vi "CurrentSwitchValues_GlobalVariable.vi"() -> ()   [LabVIEW 2018]
panel:
  out "Current Reactor":dbl
  in  "Reactor RR Array":dbl[](array[numeric])
  out "Refresh Ratio Reactor 8":dbl
  out "Refresh Ratio Reactor 7":dbl
  out "Refresh Ratio Reactor 6":dbl
  out "Refresh Ratio Reactor 5":dbl
  out "Refresh Ratio Reactor 4":dbl
  out "Refresh Ratio Reactor 3":dbl
  out "Refresh Ratio Reactor 2":dbl
  out "Refresh Ratio Reactor 1":dbl
  out "Refresh Ratio Average":dbl
  out "Number of Inflow Steps Used During Calibration":dbl
  out "30":bool
  out "29":bool
  out "28":bool
  out "27":bool
  out "26":bool
  out "25":bool
  out "24":bool
  out "23":bool
  out "22":bool
  out "21":bool
  out "20":bool
  out "19":bool
  out "18":bool
  out "17":bool
  out "16":bool
  out "15":bool
  out "14":bool
  out "13":bool
  out "12":bool
  out "11":bool
  out "10":bool
  out "9":bool
  out "8":bool
  out "7":bool
  out "6":bool
  out "5":bool
  out "4":bool
  out "3":bool
  out "2":bool
  out "1":bool
  # "The numerical indicators below record the number of inflow\nSteps used during a single dilution step during the calibration\nand the resulting refresh ratio which is achieved using this \ninflow duration. These will be set after the calibration and will\nnot be adapted thereafter. In this way they can be used as \nconstants in the following experiments."
  # "The boolean indicators are used to\nprovide global variables representing \nthe current state of each of the solenoid\nvalves."
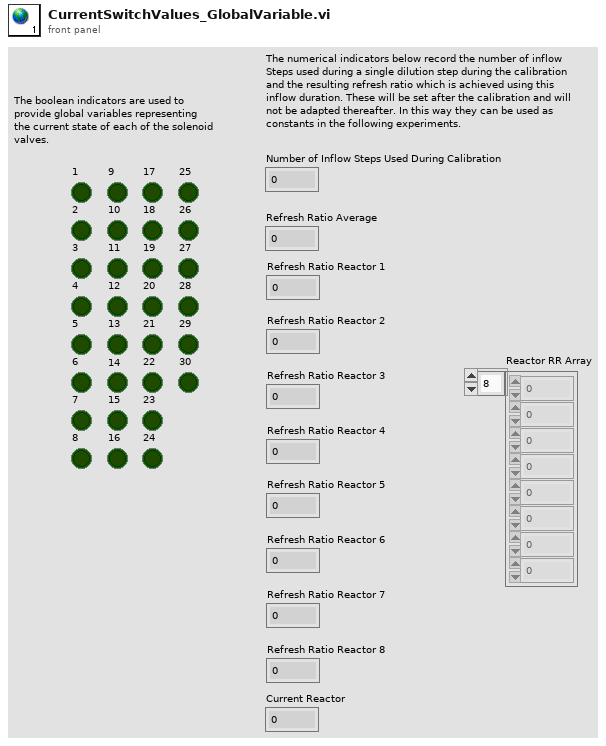
[diagram p1: front panel]
diagram:
